vi "Main.vi"() -> ()   [LabVIEW 2020]
uses:
  FSM_States.ctl
  <vilib>/Utility/miscctls.llb/LVPointTypeDef.ctl
  <vilib>/Instr/_visa.llb/VISA Configure Serial Port (Instr).vi
panel:
  out "NumOfSignal":u8
  out "Output Plot":cluster{"X2":dbl[], "Y2":dbl[]}[](graph)
  out "FSM State":T1
  in  "Cancel trigger":bool
  out "Status":string
  out "error out":errorcluster
  in  "Set Trigger":bool
  in  "Close":bool
  in  "Connect":bool
  in  "Port":refnum<visa-resource-name>
  in  "Digital channel 4":bool
  in  "Digital channel 3":bool
  in  "Digital channel 2":bool
  in  "Digital channel 1":bool
  in  "Analog channel 4":bool
  in  "Analog channel 3":bool
  in  "Analog channel 2":bool
  in  "Analog channel 1":bool
  in  "Trigger level":sgl min=0 max=24 format="%#_g V"
  in  "Trigger on channel [1-4]":enum8{"1", "2", "3", "4"}(ring)
  in  "Trigger type":T2(ring)
  # "Connection Setup"
  # "Trigger Setup"
  # "Channel to Log"
  # "Programm Status"
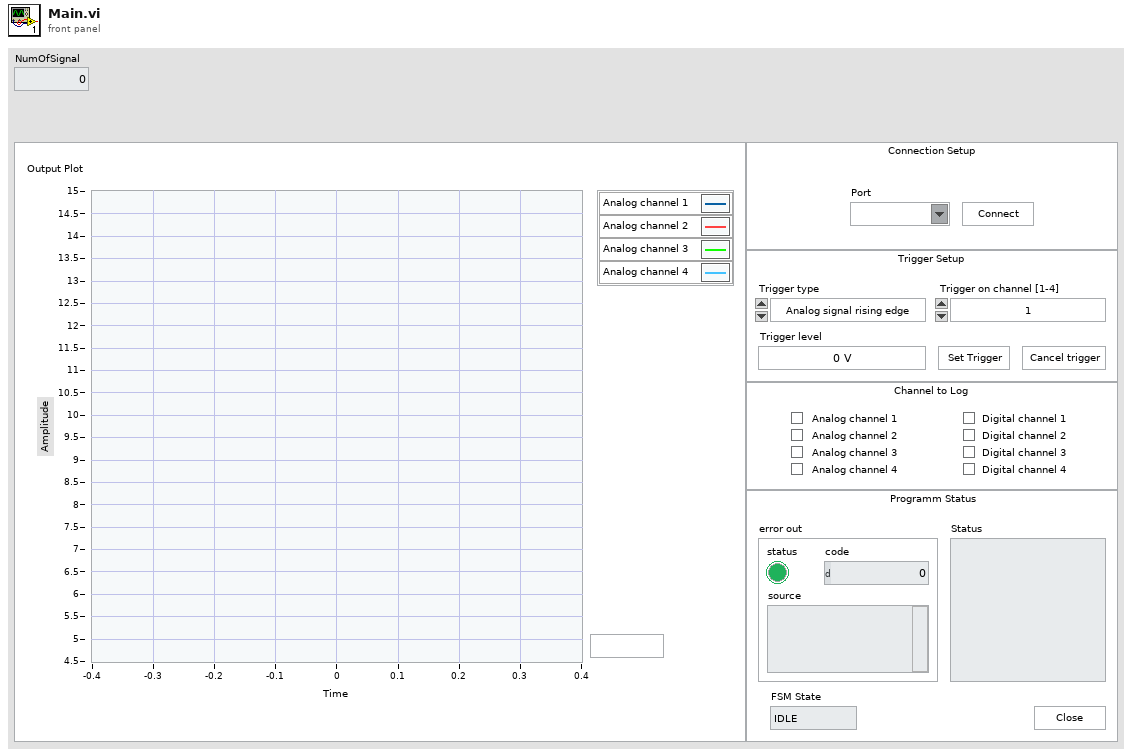
[diagram p1: front panel]
types:
  T1 = typedef "FSM_States.ctl" = enum16{"IDLE", "Read Data"}
  T2 = enum8{"Analog signal rising edge", "Analog signal falling edge", "Digital signal = 1", "Digital signal = 0"}
  T3 = typedef "LVPointTypeDef.ctl" = cluster{"Horizontal":i16, "Vertical":i16}
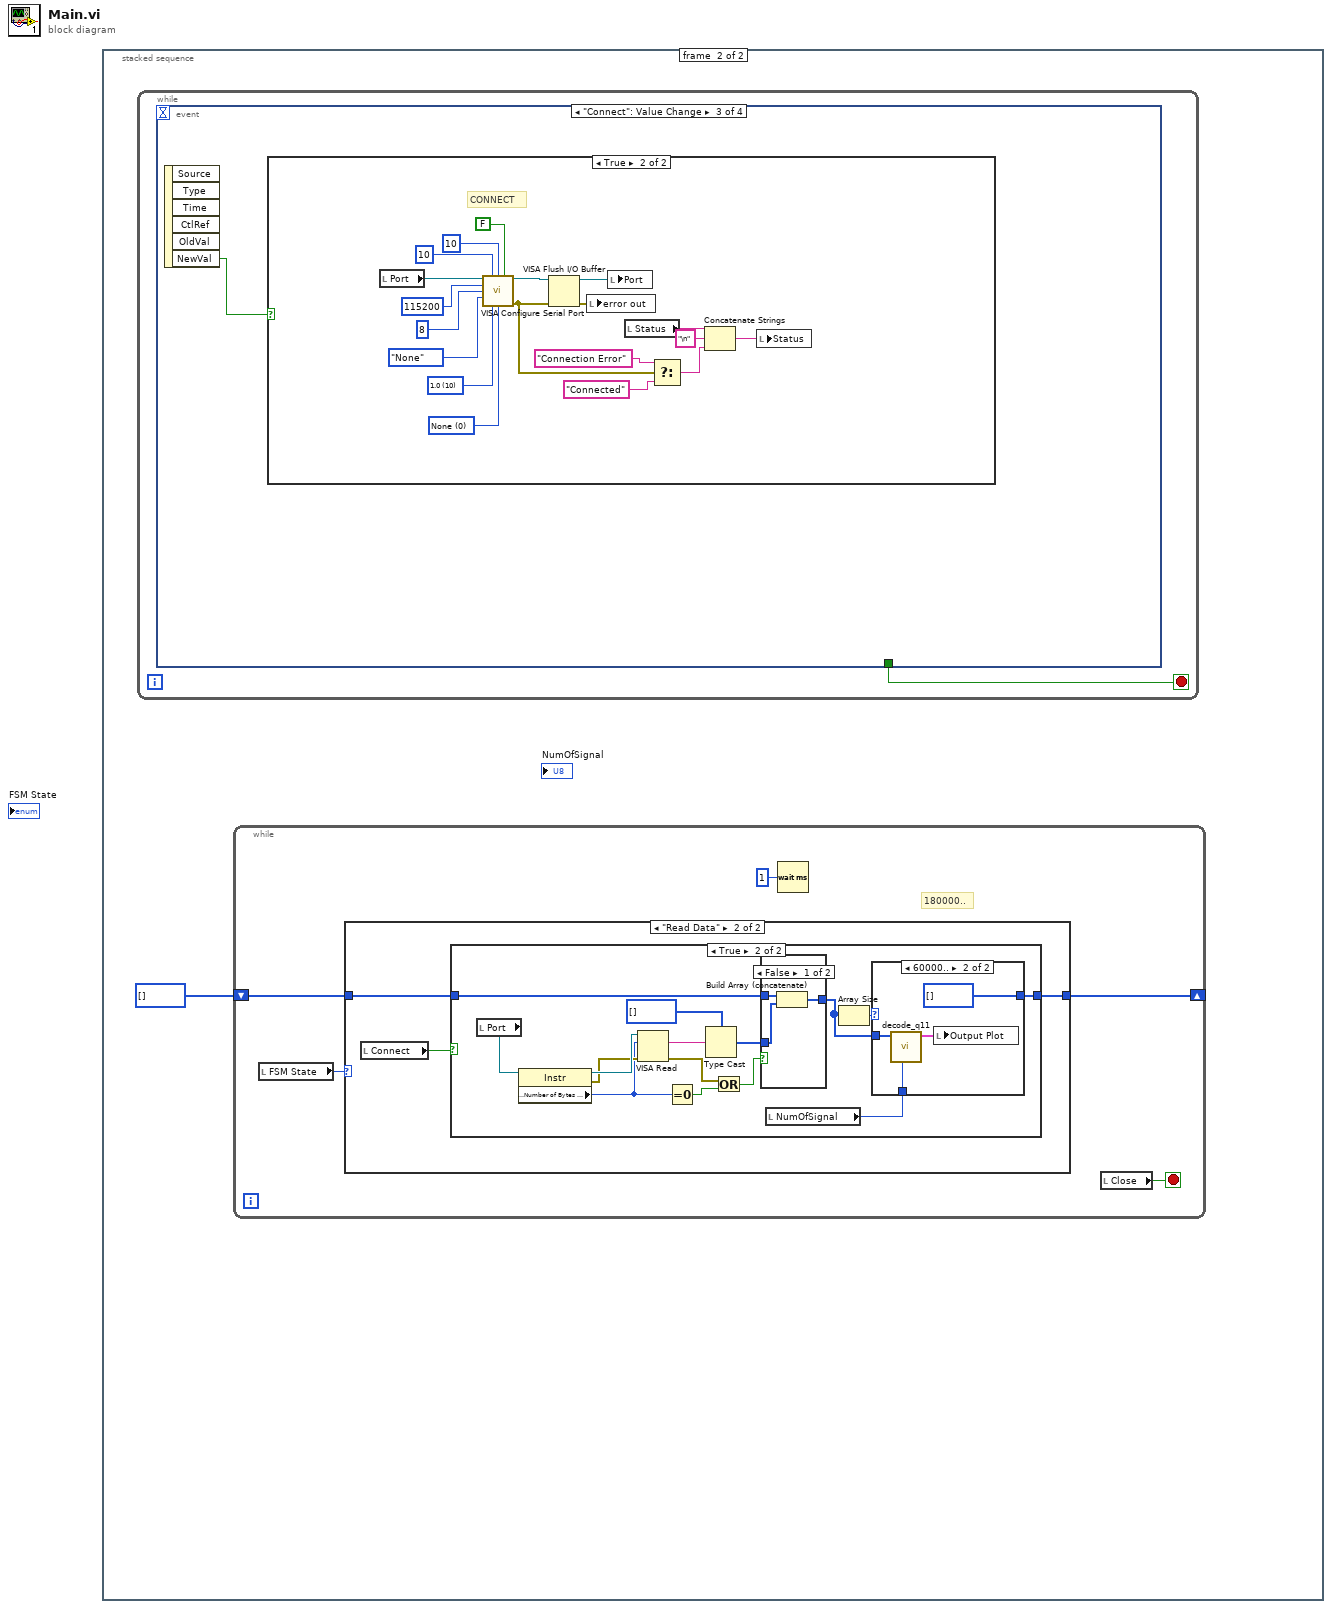
[diagram p0: block diagram]
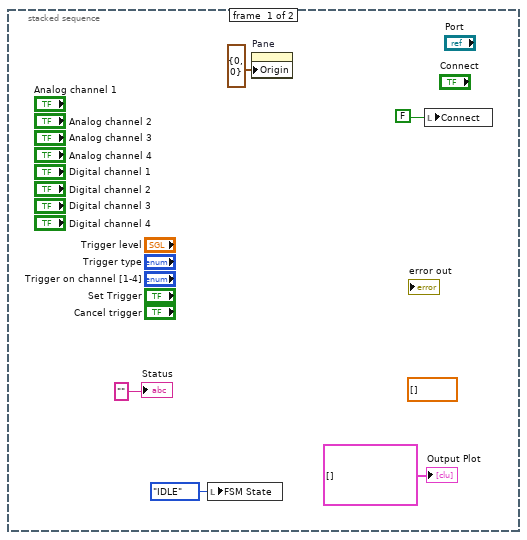
[diagram p2: hidden frame]
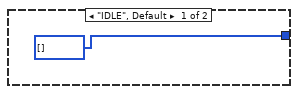
[diagram p3: hidden frame]
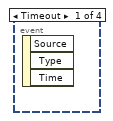
[diagram p7: hidden frame]
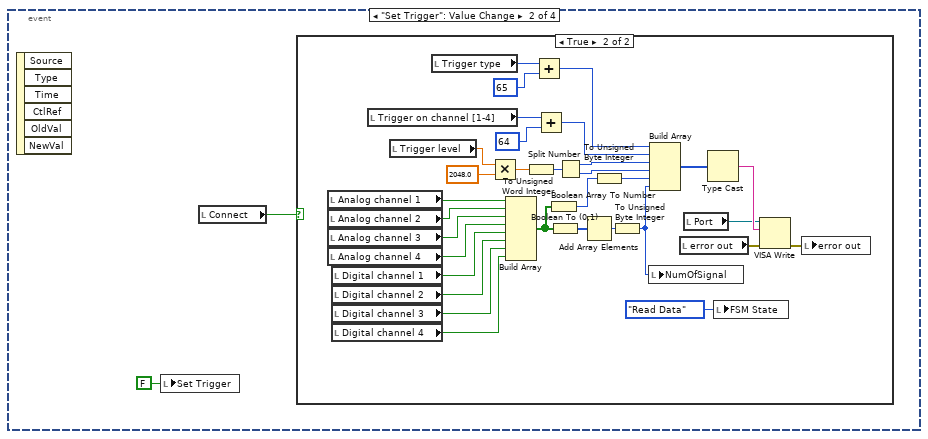
[diagram p8: hidden frame]
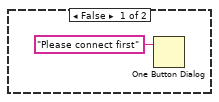
[diagram p9: hidden frame]
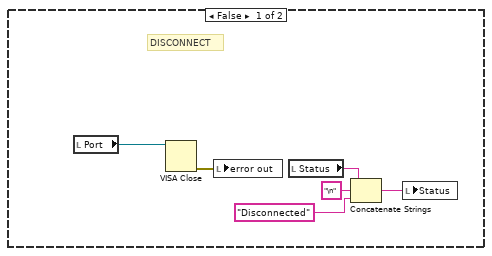
[diagram p10: hidden frame]
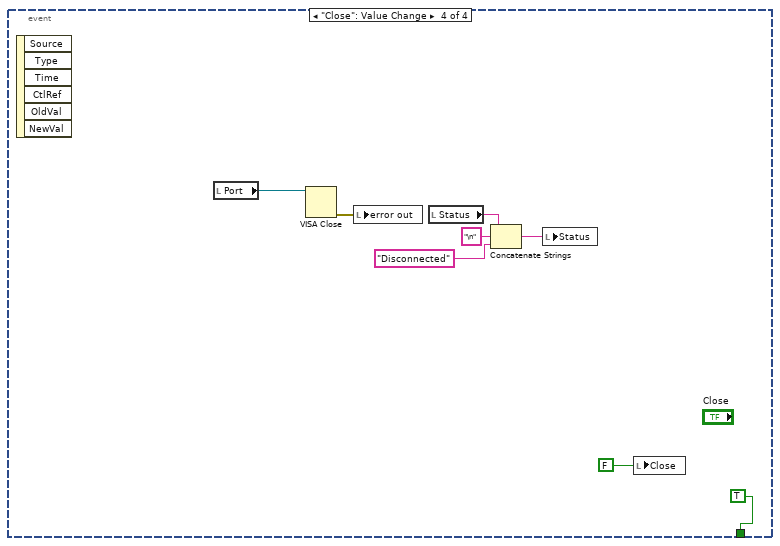
[diagram p11: hidden frame]
diagram:
  n1 = stacked-sequence {
    frame #0 {
      (unwired) dbl[] []
      n2 = local write "FSM State"(enum16{"IDLE", "Read Data"}."IDLE" ("FSM State")) -> ()
      n3 = property on="Pane" class="Pane"("Origin"=T3 {"Horizontal"=0, "Vertical"=0}) -> ()  [unwired: 2 in, 2 out]
      n4 = local write "Connect"(FALSE ("Connect")) -> ()
      "Status" <- "" ("Status")
      "Output Plot" <- cluster{"X2":dbl[], "Y2":dbl[]}[] [] ("Output Plot")
    }
    frame #1 {
      n5 = while {
        stop <- w41 stop-if-true
        n6 = event shown="[2] \"Connect\": Value Change" {
          selector: _ -> [_ _ _ _]
          dyn-events: _ -> [_ _ _ _]
          timeout: _ -> [_ _ _ _]
          tunnel: [_ _ _ TRUE ("Close")] -> w41
          event Timeout {
            n7 = event-data() -> ()  [unwired: 1 in, 3 out]
          }
          event "Set Trigger": Value Change {
            n8 = event-data() -> ()  [unwired: 1 in, 6 out]
            n9 = local write "Set Trigger"(FALSE ("Set Trigger")) -> ()
            n10 = local read "Connect"() -> (w42:bool)
            n11 = case shown="True" w42 {
              frame False {
                n12 = One Button Dialog(message="Please connect first") -> ()  [unwired: 1 in, 1 out]
              }
              frame True {
                n13 = local read "Analog channel 1"() -> (w54:bool)
                n14 = local read "Analog channel 2"() -> (w55:bool)
                n15 = local read "Analog channel 3"() -> (w56:bool)
                n16 = local read "Analog channel 4"() -> (w57:bool)
                n17 = local read "Digital channel 1"() -> (w58:bool)
                n18 = local read "Digital channel 2"() -> (w59:bool)
                n19 = local read "Digital channel 3"() -> (w60:bool)
                n20 = local read "Digital channel 4"() -> (w61:bool)
                n21 = local read "Trigger on channel [1-4]"() -> (w63:enum8{"1", "2", "3", "4"})
                n22 = local read "Trigger level"() -> (w64:sgl)
                n23 = local read "Trigger type"() -> (w62:T2)
                n24 = Multiply(x=w64, y=sgl 2048.0) -> (x*y=w65:sgl)
                n25 = Build Array(w54, w55, w56, w57, w58, w59, w60, w61) -> (w71:bool[])
                n26 = To Unsigned Word Integer(number=w65) -> (unsigned 16bit integer=w66:u16)
                n27 = Add(x=w62, y=u8 65) -> (x+y=w67:u8)
                n28 = Add(x=w63, y=u8 64) -> (x+y=w68:u8)
                n29 = Boolean Array To Number(Boolean array=w71) -> (number=w73:u32)
                n30 = Boolean To (0,1)(Boolean=w71) -> (0, 1=w72:i16[])
                n31 = Split Number(x=w66) -> (hi(x)=w69:u8, lo(x)=w70:u8)
                n32 = Add Array Elements(numeric array=w72) -> (sum=w74:i16)
                n33 = To Unsigned Byte Integer(number=w73) -> (unsigned 8bit integer=w46:u8)
                n34 = To Unsigned Byte Integer(number=w74) -> (unsigned 8bit integer=w45:u8)
                n35 = local write "NumOfSignal"(w45) -> ()
                n36 = Build Array(w67, w68, w69, w70, w46, w45) -> (w75:u8[])
                n37 = local read "error out"() -> (w49:errorcluster)
                n38 = local read "Port"() -> (w50:refnum<visa-resource-name>)
                n39 = Type Cast(x=w75) -> (*(type *) &x=w76:string)  [unwired: 1 in]
                n40 = local write "FSM State"(FSM_States."Read Data" ("FSM State")) -> ()
                n41 = VISA Write(VISA resource name=w50, write buffer=w76, error in (no error)=w49) -> (error out=w48:errorcluster)  [unwired: 2 out]
                n42 = local write "error out"(w48) -> ()
              }
            }
          }
          event "Connect": Value Change {
            n43 = event-data() -> ("NewVal"=w77:bool)  [unwired: 1 in, 5 out]
            n44 = case shown="True" w77 {
              frame False {
                # "DISCONNECT"
                n45 = local read "Port"() -> (w82:refnum<visa-resource-name>)
                n46 = VISA Close(VISA resource name=w82) -> (error out=w83:errorcluster)  [unwired: 1 in]
                n47 = local write "error out"(w83) -> ()
                n48 = local read "Status"() -> (w78:string)
                n49 = Concatenate Strings(w78, "\n" ("string"), "Disconnected" ("string")) -> (w81:string)
                n50 = local write "Status"(w81) -> ()
              }
              frame True {
                w85 = u16 0 items=["None", "XON/XOFF", "RTS/CTS", "XON/XOFF & RTS/CTS", "DTR/DSR", "XON/XOFF & DTR/DSR"] ("flow control (0:none)")
                w86 = u16 10 items=["1.0"=10, "1.5"=15, "2.0"=20] ("stop bits (10: 1 bit)")
                # "CONNECT"
                n51 = local read "Port"() -> (w100:refnum<visa-resource-name>)
                n52 = call-poly "VISA Configure Serial Port"("VISA resource name"=w100, "timeout (10sec)"=u32 10, "termination char\n(0xA = '\\n' = LF)"=u8 10 ("termination char\n(0xA = '\\n' = LF)"), "Enable Termination\nChar (T)"=FALSE ("Enable Termination\nChar (T)"), "baud rate (9600)"=u32 115200, "data bits (8)"=u16 8, "parity (0:none)"=enum16{"None", "Odd", "Even", "Mark", "Space"}."None", "stop bits (10: 1 bit)"=w86, "flow control (0:none)"=w85) -> ("VISA resource name out"=w92:refnum<visa-resource-name>, "error out"=w91:errorcluster)  [unwired: 5 in]
                n53 = VISA Flush I/O Buffer(VISA resource name=w92, error in (no error)=w91) -> (VISA resource name out=w90:refnum<visa-resource-name>, error out=w89:errorcluster)  [unwired: 1 in]
                n54 = local write "error out"(w89) -> ()
                n55 = local write "Port"(w90) -> ()
                n56 = local read "Status"() -> (w99:string)
                n57 = Select(t="Connection Error" ("string"), s=w91, f="Connected" ("string")) -> (s? t:f=w94:string)
                n58 = Concatenate Strings(w99, "\n" ("string"), w94) -> (w98:string)
                n59 = local write "Status"(w98) -> ()
              }
            }
          }
          event "Close": Value Change {
            n60 = event-data() -> ()  [unwired: 1 in, 6 out]
            n61 = local read "Port"() -> (w109:refnum<visa-resource-name>)
            n62 = VISA Close(VISA resource name=w109) -> (error out=w110:errorcluster)  [unwired: 1 in]
            n63 = local write "error out"(w110) -> ()
            n64 = local read "Status"() -> (w107:string)
            n65 = Concatenate Strings(w107, "\n" ("string"), "Disconnected" ("string")) -> (w108:string)
            n66 = local write "Status"(w108) -> ()
            n67 = local write "Close"(FALSE ("Close")) -> ()
          }
        }
      }
      n68 = while {
        shift-right: [w8] -> _
        shift-left: u8[] [] -> [w9]
        stop <- w11 stop-if-true
        # "180000.."
        n69 = local read "FSM State"() -> (w10:T1)
        n70 = case shown="\"Read Data\"" w10 {
          tunnel: w9 -> [_ w14]
          tunnel: [u8[] [] w13] -> w8
          frame "IDLE", Default {
          }
          frame "Read Data" {
            n71 = local read "Connect"() -> (w15:bool)
            n72 = case shown="True" w15 {
              tunnel: w14 -> [w16 w30]
              tunnel: [w16 w18] -> w13
              frame False {
              }
              frame True {
                n73 = local read "Port"() -> (w28:refnum<visa-resource-name>)
                n74 = property class="Instr"(reference=w28) -> (reference out=w27:refnum<visa-resource-name>, error out=w26:errorcluster, "Serial Settings:Number of Bytes at Serial Port"=w25:u32)  [unwired: 1 in]
                n75 = VISA Read(VISA resource name=w27, byte count=w25, error in (no error)=w26) -> (read buffer=w31:string, error out=w24:errorcluster)  [unwired: 2 out]
                n76 = Equal To 0?(x=w25) -> (x = 0?=w23:bool)
                n77 = Type Cast(type=u8[] [], x=w31) -> (*(type *) &x=w29:u8[])
                n78 = Or(x=w24, y=w23) -> (x .or. y?=w22:bool)
                n79 = case shown="False" w22 {
                  tunnel: w30 -> [w39 w40]
                  tunnel: w29 -> [w38 _]
                  tunnel: [w37 w40] -> w19
                  frame False {
                    n80 = Build Array (concatenate)(w39, w38) -> (w37:u8[])
                  }
                  frame True {
                  }
                }
                n81 = local read "NumOfSignal"() -> (w17:u8)
                n82 = Array Size(array=w19) -> (size(s)=w20:i32)
                n83 = case shown="60000.." w20 {
                  tunnel: w19 -> [w32 w34]
                  tunnel: [w32 u8[] []] -> w18
                  tunnel: w17 -> [_ w35]
                  frame 0, Default {
                  }
                  frame 60000.. {
                    n84 = call "decode_q11.vi"("NumOfSignal"=w35, "Input Array u8"=w34) -> ("Output Plot"=w36:cluster{"X2":dbl[], "Y2":dbl[]}[])  [unwired: 9 in]
                    n85 = local write "Output Plot"(w36) -> ()
                  }
                }
              }
            }
          }
        }
        n86 = Wait (ms)(milliseconds to wait=u32 1) -> ()  [unwired: 1 out]
        n87 = local read "Close"() -> (w11:bool)
      }
    }
  }
